vi "GOOP400_ConfigurationMemory.vi"(1 "OptionsIn":T1, 5 "error in (no error)":errorcluster, 6 "Action":enum16{"Read", "Load", "Save"}(ring)) -> (15 "OptionsOut":T1, 19 "error out":errorcluster)   [LabVIEW 2020]
uses:
  <resource>/Framework/Providers/Open_GDS/ClassProviders/Provider_EndevoGOOP400/GOOP400_SubVIs/GOOP400_Options.ctl
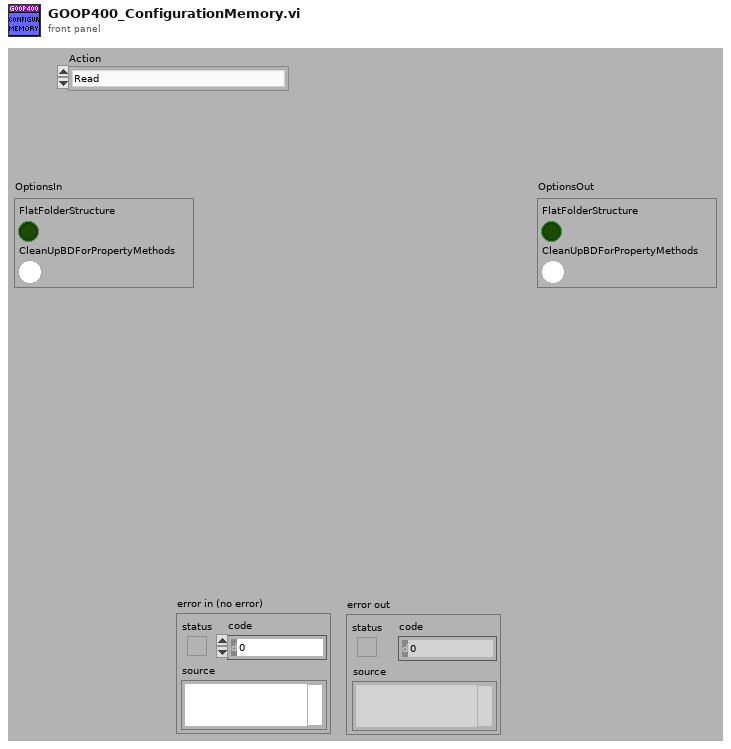
[diagram p1: front panel]
types:
  T1 = typedef "GOOP400_Options.ctl" = cluster{"FlatFolderStructure":bool, "CleanUpBDForPropertyMethods":bool}
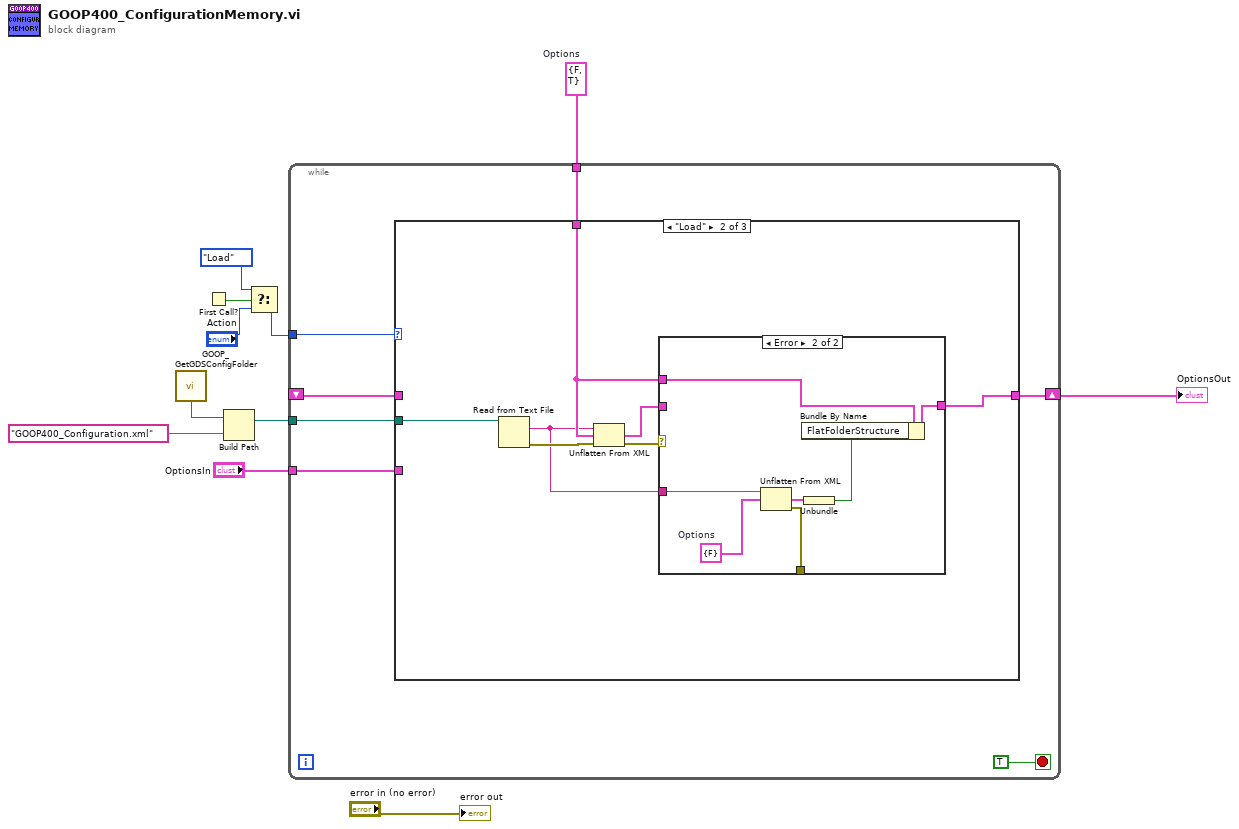
[diagram p0: block diagram]
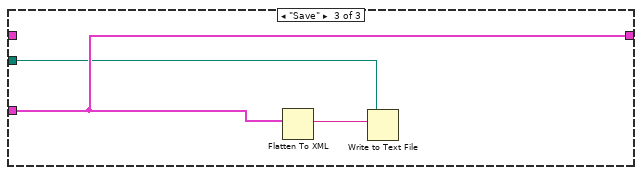
[diagram p4: hidden frame]
diagram:
  w1 = T1 {"FlatFolderStructure"=FALSE, "CleanUpBDForPropertyMethods"=TRUE}  # Options
  n1 = call <resource>:"GOOP_GetGDSConfigFolder.vi"() -> ("GDSFolderPath"=w10:path)
  n2 = First Call?() -> (First Call?: T/F=w7:bool)
  n3 = Build Path(base path=w10, name or relative path="GOOP400_Configuration.xml") -> (appended path=w9:path)
  n4 = Select(t=enum16{"Read", "Load", "Save"}."Load", s=w7, f="Action") -> (s? t:f=w5:enum16{"Read", "Load", "Save"})
  n5 = while {
    tunnel: w5 -> [w18]
    tunnel: w9 -> [w17]
    tunnel: w1 -> [w16]
    shift-right: [w14] -> w8
    shift-left: _ -> [w13]
    tunnel: "OptionsIn" -> [w12]
    stop <- TRUE stop-if-true
    n6 = case shown="\"Load\"" w18 {
      tunnel: w17 -> [_ w23 w35]
      tunnel: w16 -> [_ w22 _]
      tunnel: [w19 w21 w36] -> w14
      tunnel: w13 -> [w19 _ _]
      tunnel: w12 -> [_ _ w36]
      frame "Read", Default {
      }
      frame "Load" {
        n7 = Read from Text File(file (use dialog)=w23) -> (text=w20:string, error out=w24:errorcluster)  [unwired: 3 in, 2 out]
        n8 = Unflatten From XML(xml string=w20, type=w22, error in (no error)=w24) -> (value=w26:T1, error out=w25:errorcluster)
        n9 = case shown="Error" w25 {
          tunnel: w26 -> [w27 _]
          tunnel: [w27 w30] -> w21
          tunnel: w22 -> [_ w34]
          tunnel: w20 -> [_ w33]
          tunnel: [_ w28] -> _
          frame No Error {
          }
          frame Error {
            w32 = cluster{"FlatFolderStructure":bool} {"FlatFolderStructure"=FALSE}  # Options
            n10 = Unflatten From XML(xml string=w33, type=w32) -> (value=w31:cluster{"FlatFolderStructure":bool}, error out=w28:errorcluster)  [unwired: 1 in]
            n11 = Unbundle(w31) -> ("FlatFolderStructure"=w29:bool)
            n12 = Bundle By Name(cluster=w34, "FlatFolderStructure"=w29) -> (w30:T1)
          }
        }
      }
      frame "Save" {
        n13 = Flatten To XML(6:w36) -> (2:w37:string)
        n14 = Write to Text File(file (use dialog)=w35, text=w37) -> ()  [unwired: 2 in, 3 out]
      }
    }
  }
  "OptionsOut" <- w8
  "error out" <- "error in (no error)"
